vi "String.vi"() -> ()   [LabVIEW 2022 SP3]
panel:
  out "decimal integer string":string
  out "number":u32
  out "concatenated string":string
  out "substring":string
  out "length 2":i32
  out "length":i32
  out "String 2":string
  out "String":string
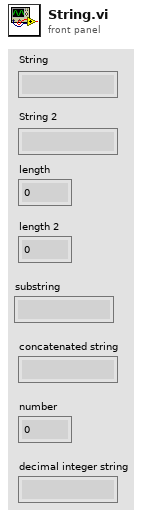
[diagram p1: front panel]
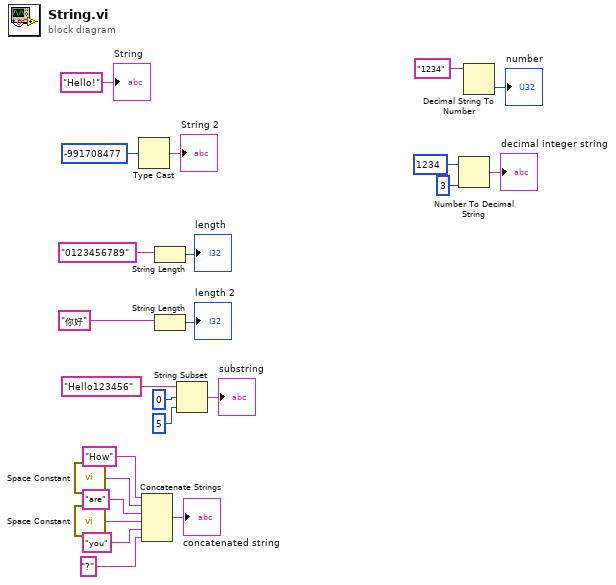
[diagram p0: block diagram]
diagram:
  n1 = call <vilib>:"Space Constant.vi"() -> ("String"=w10:string)
  n2 = call <vilib>:"Space Constant.vi"() -> ("String"=w8:string)
  n3 = Type Cast(x=-991708477) -> (*(type *) &x=→"String 2":string)  [unwired: 1 in]
  n4 = Concatenate Strings("How", w10, "are", w8, "you", "?") -> (→"concatenated string":string)
  n5 = String Length(string="0123456789") -> (length=→"length":i32)
  n6 = String Length(string="你好") -> (length=→"length 2":i32)
  n7 = String Subset(string="Hello123456", offset (0)=0, length (rest)=5) -> (substring=→"substring":string)
  n8 = Number To Decimal String(number=1234, width (-)=i16 3) -> (decimal integer string=→"decimal integer string":string)
  n9 = Decimal String To Number(string="1234") -> (number=→"number":i32)  [unwired: 2 in, 1 out]
  "String" <- "Hello!"
